vi "Read all custom data.vi"(8 "error in (no error)":errorcluster, 11 "img":T1) -> (0 "error out":errorcluster, 1 "Custom Data":string[](array[string]), 2 "Keys":string[](array[string]), 3 "Image (duplicate)":T1)   [LabVIEW 2013]
doc: "This .vi returns all custom data stored in the image buff."
uses:
  <vilib>/vision/Image Controls.llb/IMAQ Image.ctl
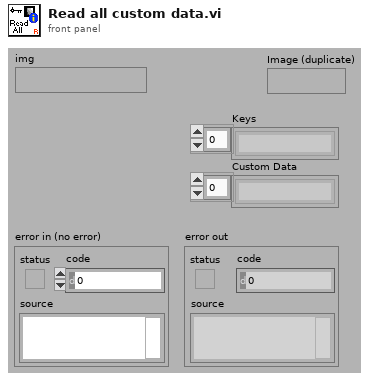
[diagram p1: front panel]
types:
  T1 = typedef "IMAQ Image.ctl" = refnum<image>
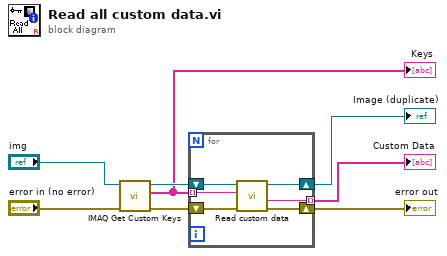
[diagram p0: block diagram]
diagram:
  n1 = call "IMAQ Get Custom Keys"("error in (no error)"="error in (no error)", "Image"="img") -> ("error out"=w5:errorcluster, "Keys"=w4:string[], "Image (duplicate)"=w7:T1)  [unwired: 7 out]
  "Keys" <- w4
  n2 = for {
    shift-right: [w13] -> w1
    shift-left: w7 -> [w14]
    tunnel: w4 -> [w12] mode=indexing
    tunnel: [w9] -> w3 mode=indexing
    shift-right: [w10] -> w2
    shift-left: w5 -> [w11]
    n3 = call "Read custom data.vi"("error in"=w11, "Key"=w12, "Image"=w14) -> ("error out"=w10:errorcluster, "Custom Data Out"=w9:string, "Image (duplicate)"=w13:T1)  [unwired: 6 in]
  }
  "error out" <- w2
  "Custom Data" <- w3
  "Image (duplicate)" <- w1
